vi "FestoCPX.WaitForInit.vi"   [LabVIEW 2016]
uses:
  FestoCPX.State.ctl
  FestoCPX.Global.vi
  Global/ApplicationGlobal.vi
types:
  T1 = typedef "FestoCPX.State.ctl" = enum16{"First", "Error", "Init", "Run"}
  T2 = typedef "FestoCPX.Data.Status.ctl" = cluster{"State":T1, "Conn":refnum<k5>, "TS":timestamp}
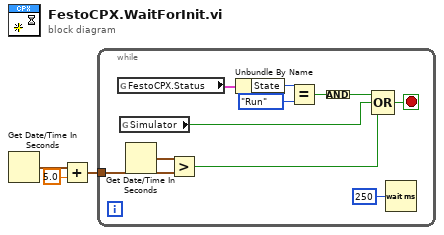
[diagram p0: block diagram]
diagram:
  n1 = Get Date/Time In Seconds() -> (seconds since 1Jan1904=w3:timestamp)
  n2 = Add(x=w3, y=5.0) -> (x+y=w1:timestamp)
  n3 = while {
    tunnel: w1 -> [w8]
    stop <- w4 stop-if-true
    n4 = global read "FestoCPX.Global.vi" "FestoCPX.Status"() -> (w14:T2)
    n5 = global read "ApplicationGlobal.vi" "Simulator"() -> (w5:bool)
    n6 = Get Date/Time In Seconds() -> (seconds since 1Jan1904=w7:timestamp)
    n7 = Greater?(x=w7, y=w8) -> (0:w6:bool)
    n8 = Unbundle By Name(w14) -> ("State"=w13:T1)
    n9 = Equal?(x=w13, y=FestoCPX.State."Run") -> (x = y?=w11:bool)
    n10 = Compound Arithmetic op=AND(w11) -> (w10:bool)
    n11 = Compound Arithmetic op=OR(w10, w5, w6) -> (w4:bool)
    n12 = Wait (ms)(milliseconds to wait=u32 250) -> ()  [unwired: 1 out]
  }
